vi "connect to nosams db.vi"() -> ()   [LabVIEW 2013]
doc: "This example shows three different methods available to connect to a database: \n\n1) An ODBC data source name (DSN) that has been created from the Control Panel with the Data Sources (ODBC) utility. When you installed the LabVIEW Database Tools, a DSN named LabVIEW was automatically created. This LabVIEW DSN uses the Microsoft Access Driver and refers to the database file labview.mdb in the examples\\database directory.\n\n2) A universal data link (UDL) file created from the LabVIEW Tools>>Create Data Link option. When you installed the LabVIEW Database Tools, the LabVIEW.udl file in the examples\\database directory and UDL file extensions were registered in the Windows registry. \n\n3) A dialog prompt can be used to select the data link properties for a database connection."
uses:
  <vilib>/addons/database/Connection.llb/DB Tools Open Connec (String).vi
  <vilib>/addons/database/NI_Database_API.lvlib
panel:
  out "Connection Succeeded?":bool
  # "This VI shows three different methods available to connect to a database: an ODBC data source name (DSN), universal data link (UDL) file, or using a dialog prompt."
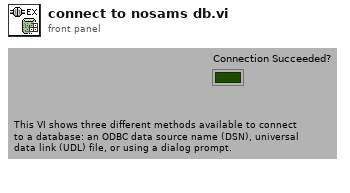
[diagram p1: front panel]
types:
  T1 = typedef "NI_Database_API.lvlib/Conn ObjectReference.ctl" = refnum<k1>
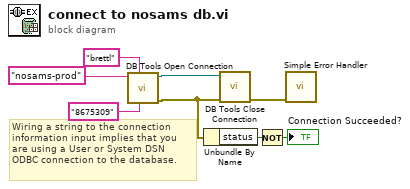
[diagram p0: block diagram]
diagram:
  # "Wiring a string to the connection \ninformation input implies that you \nare using a User or System DSN \nODBC connection to the database."
  n1 = call-poly <vilib>:"DB Tools Open Connection.vi"("password"="8675309", "userID"="brettl", "connection information"="nosams-prod") -> ("error out"=w4:errorcluster, "connection reference"=w7:T1)  [unwired: 5 in]
  n2 = Unbundle By Name(w4) -> ("status"=w5:bool)
  n3 = call <vilib>:"DB Tools Close Connection.vi"("error in (no error)"=w4, "connection reference"=w7) -> ("error out"=w8:errorcluster)  [unwired: 5 in]
  n4 = Not(x=w5) -> (.not. x?=→"Connection Succeeded?":bool)
  n5 = call <vilib>:"Simple Error Handler.vi"("error in (no error)"=w8) -> ()  [unwired: 4 in, 5 out]
